vi "Read Response.vi"(8 "error in (no error)":errorcluster, 11 "VISA resource name":refnum<visa-resource-name>) -> (0 "error out":errorcluster, 2 "Confirmation Response":string, 3 "VISA resource name out":refnum<visa-resource-name>)   [LabVIEW 2015, in "Micron Optics sm130.lvlib"]
doc: "Reads the response from the instrument. Error responses will be passes through the error cluster. Confirmation response string output is for convinience and can be ignored."
uses:
  Micron Optics sm130.lvlib
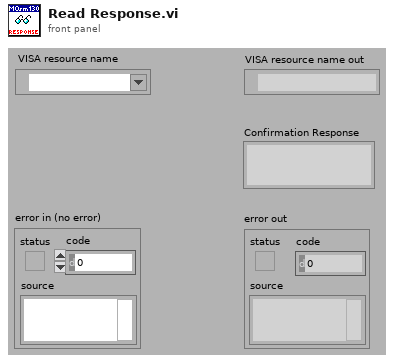
[diagram p1: front panel]
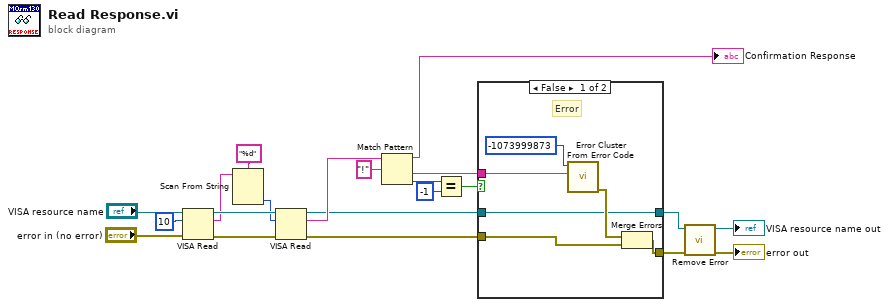
[diagram p0: block diagram]
diagram:
  n1 = VISA Read(VISA resource name="VISA resource name", byte count=u32 10, error in (no error)="error in (no error)") -> (VISA resource name out=w20:refnum<visa-resource-name>, read buffer=w16:string, error out=w21:errorcluster)  [unwired: 1 out]
  n2 = Scan From String(format string="%d", input string=w16) -> (output 1=w15:i32)  [unwired: 3 in, 3 out]
  n3 = VISA Read(VISA resource name=w20, byte count=w15, error in (no error)=w21) -> (VISA resource name out=w7:refnum<visa-resource-name>, read buffer=w14:string, error out=w8:errorcluster)  [unwired: 1 out]
  n4 = Match Pattern(string=w14, regular expression="!") -> (before substring=→"Confirmation Response":string, after substring=w9:string, offset past match=w12:i32)  [unwired: 1 in, 1 out]
  n5 = Equal?(x=w12, y=-1) -> (x = y?=w10:bool)
  n6 = case shown="False" w10 {
    tunnel: w9 -> [w26 _]
    tunnel: w8 -> [w24 w28]
    tunnel: w7 -> [w23 w29]
    tunnel: [w23 w29] -> w1
    tunnel: [w22 w28] -> w4
    frame False {
      # "Error"
      n7 = call <vilib>:"Error Cluster From Error Code.vi"("error message (\"\")"=w26, "error code (0)"=-1073999873) -> ("error out"=w25:errorcluster)  [unwired: 7 in]
      n8 = Merge Errors(w25, w24) -> (w22:errorcluster)
    }
    frame True {
      # "No Error"
    }
  }
  n9 = call "Remove Error.vi"("error in (no error)"=w4, "VISA resource name"=w1) -> ("error out"=→"error out":errorcluster, "VISA resource name out"=→"VISA resource name out":refnum<visa-resource-name>)  [unwired: 8 in]
